vi "get_firmware.vi"(6 "timeout (25000ms)":i32=25000, 8 "error in (no error)":errorcluster, 9 "firmware information":string(combo)="variables", 11 "daemon reference in":refnum<k5>) -> (0 "error out":errorcluster, 2 "object names":string[](array[string]), 3 "daemon reference out":refnum<k5>, 5 "command out":string="random")   [LabVIEW 2017]
doc: "<b>Command: </b>\"get_firmware\"\n\n<b>Description: </b> This command extracts the available JSON elements which correspond to the desired type (e.g. variables for peek/poke).\n\n<b>Parameters: </b> \n\n 1. Firmware Information (\"variables\" / \"errors\" / \"typedefs\" / \"functions\" / \"enums\")\n____________________________________________\nDIPC 692 Daemon API 10.0.0.1\nSam Tee - Dyson Technology Ltd\nCopyright (c) 2024, Dyson Technology Ltd"
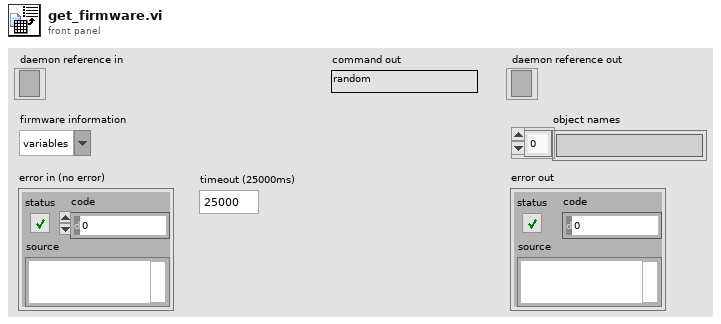
[diagram p1: front panel]
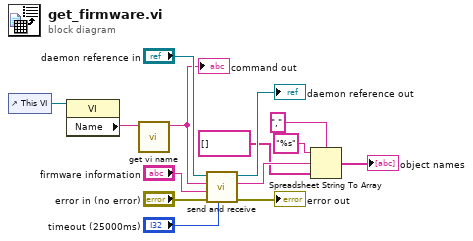
[diagram p0: block diagram]
diagram:
  n1 = control-ref of="This VI"() -> (w9:refnum<vi>)
  n2 = property class="VI"(reference=w9) -> ("Name"=w8:string)  [unwired: 1 in, 2 out]
  n3 = call "get vi name.vi"("library.lvlib:name.vi"=w8) -> ("vi name"=w7:string)  [unwired: 10 in]
  "command out" <- w7
  n4 = call "send and receive.vi"("timeout (25000ms)"="timeout (25000ms)", "error in (no error)"="error in (no error)", "data"="firmware information", "command"=w7, "daemon reference in"="daemon reference in") -> ("error out"=→"error out":errorcluster, "response"=w6:string, "daemon reference out"=→"daemon reference out":refnum<k5>)  [unwired: 4 in]
  n5 = Spreadsheet String To Array(delimiter (Tab)=",", format string="%s", spreadsheet string=w6, array type (2D Dbl)=string[] []) -> (array=→"object names":string[])
